vi "Advanced Serial Write and Read - Black Magic Voodo.vi"(0 "VISA resource name":refnum<visa-resource-name>="COM11", 13 "string to write":string="*IDN?", 17 "write":bool=TRUE, 26 "read":bool=TRUE) -> (20 "read string":string)   [LabVIEW 2010]
doc: "The Advanced Serial Read and Write example performs a Serial Port Read, a Serial Port Write, or a combination of these actions while setting some advanced serial features like buffer size, termination characters, and XON/XOFF flow control. The user selects the actions (read or write) on the front panel. If both are selected, the VI will write the data first, read the data and then close the VISA session that is opened to the port. \n\nThe parameters set for the serial port must match the parameters of the connected instrument or device. In this example, the bytes to read parameter specifies the number of bytes that the serial port reads. If there were more bytes at the port than the number specified in bytes to read, those bytes would not be read. Also, if you specify to read more bytes than the number of bytes actually read, you might receive a timeout error message.\n\nINSTRUCTIONS:\n1) Select the serial resource and configuration parameters (baud rate, data bits, parity, stop bits, flow control).\n2) Termination character can be enabled and set. Also, set the required input buffer size prior to running the example.\n3) Select the operations to be performed. \n4) Connect the serial port to your device. If no device is available, perform a loopback test by doing one of the following. Short pins 2 and 3 on a RS-232 cable or short pin 4 to pin 8 and pin 5 to pin 9 on a RS-485/422 cable. \n5) Run the VI to see the data read. (The \"read string\" will match the \"string to write\" if a loopback test was performed.)\n\nThis example exposes several advanced features that you may need for your application. Not all applications need all the features shown in this example. The input buffer size is likely an important setting that you want to control in your application. This example expands upon the flow control option for XON and XOFF, allowing the user to choose those control characters. The timeout parameter has been brought to the front panel so a user can specify the time period the VISA Read will wait for the number of bytes to read before timing out. Also, the user has several controls for the termination character, which is discussed later.\n\nNote that you can press the write and read buttons and change the bytes to read parameters on the fly, while the example is running. However, you must stop the example to change the other configuration parameters after the example has started running, and then run again.\n\nSet the I/O buffer size slightly higher the amount of data you expect to receive. This is very important for applications that don't use flow control, as you may lose characters if the receive buffer overflows.\n\nSetting the timeout period ensures that the operation returns with a timeout error if the operation cannot be performed in the specified time period. \n\nSome devices require a termination character in order to identify the end of command strings. Some devices send a termination character to signify the end of data to be read. \n\nThis example shows how you can end the Read operation once a termination character is detected in the buffer and/or append a termination character at the end of the Write data. To enable the Read to end on a termination character, use the VISA Configure Serial Port or use the VISA Properties Serial End Mode for Reads, Termination Character Enable, and Termination Character. To end the Write with a termination character, use the VISA Properties Serial End Mode for Writes, the Send End Enable, and Termination Character. In this example, the same termination character is used for both the Read and the Write. You can specify two different characters for your application, if desired.\n\nYour application may require specific characters for the XON/XOFF Flow Control. You can specify these characters with the VISA Properties Flow Control XOFF Character and Flow Control XON Character. Note that if the standard XON and XOFF characters are used, then decimal 17 and 19 are unavailable for data values. Remember that using flow control and setting an adequate buffer size allow you to prevent buffer overflows."
uses:
  <vilib>/Instr/_visa.llb/VISA Configure Serial Port (Instr).vi
panel:
  in  "String":string="(RS232(Sources (\"CO2B um/m\" \"H2OB mm/m\"  \"Integral\" \"Peak\" \"P kPa\" \"T C\" ))) "
  out "iteration":dbl
  out "actual bytes read":u32
  in  "stop":bool
  # "Select the serial resource and the operations to be performed.  If all are selected, the VI will write the data first, read data and then close the VISA session that is opened to the port.  This VI will wait until the specified number of bytes is received at the port, until the timeout period is met, or until a termination character is received.  The default termination character in this example is the Line Feed ( ASCII 0xA, '\\n' ).  Also, set the required input buffer size prior to running the example.\nNote: The example loops until the STOP button is pressed."
  # "For additional information select File >> VI Properties >> Documentation"
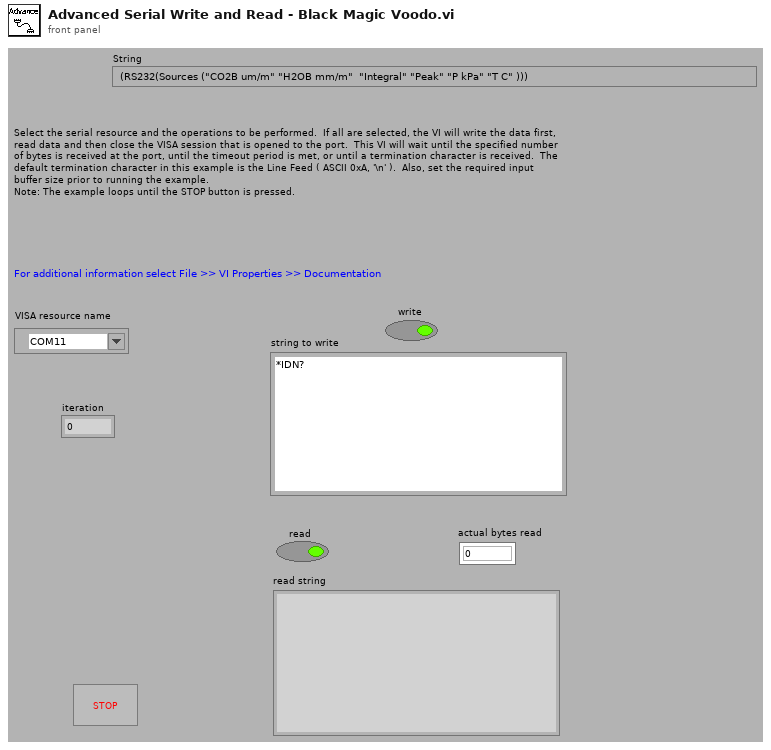
[diagram p1: front panel]
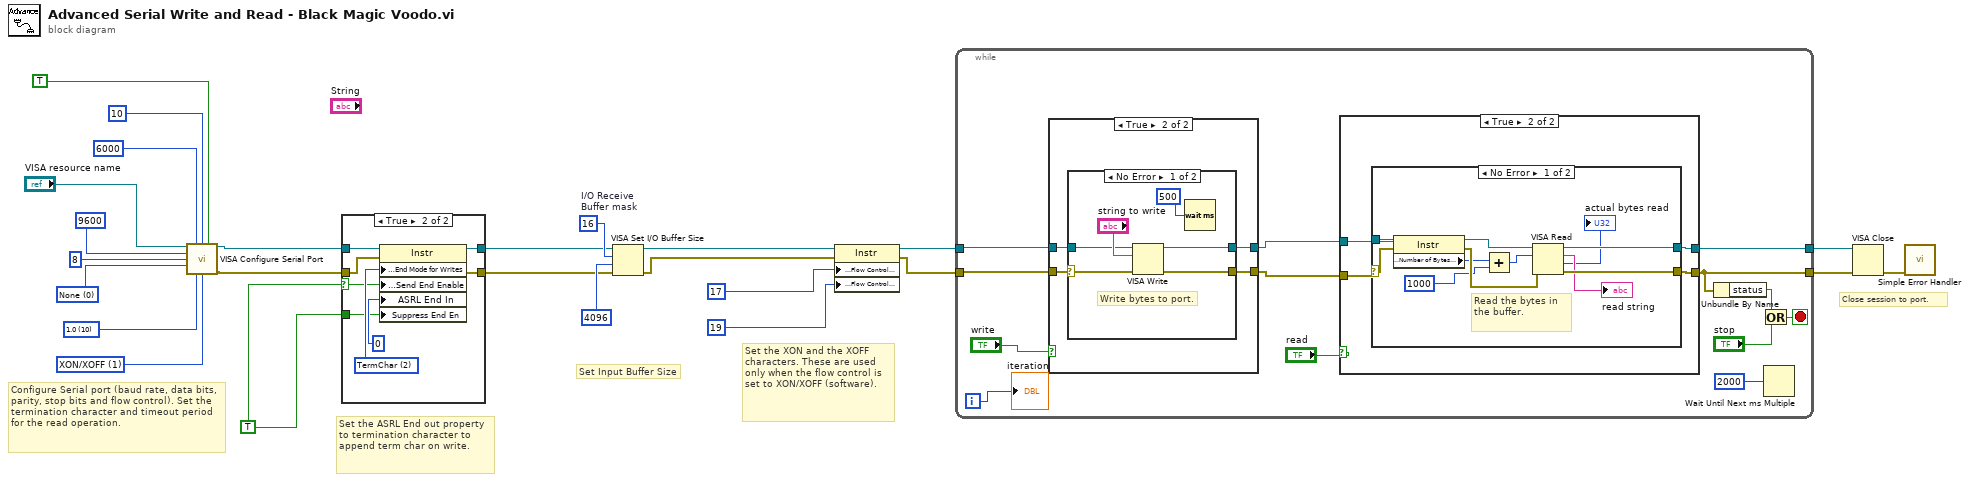
[diagram p0: block diagram]
diagram:
  w1 = TRUE ("End write with termination character?")
  w15 = u16 1 items=["None"=0, "XON/XOFF"=1, "RTS/CTS"=2, "DTR/DSR"=4] ("flow control")
  w21 = u16 10 items=["1.0"=10, "1.5"=15, "2.0"=20] ("stop bits")
  w22 = u16 0 items=["None", "Odd", "Even", "Mark", "Space"] ("parity")
  w18 = u16 16  # I/O Receive Buffer mask
  # "Set the XON and the XOFF characters. These are used only when the flow control is set to XON/XOFF (software)."
  # "Configure Serial port (baud rate, data bits, parity, stop bits and flow control). Set the termination character and timeout period for the read operation."
  # "Set Input Buffer Size"
  # "Set the ASRL End out property to termination character to append term char on write."
  # "Close session to port."
  n1 = call-poly "VISA Configure Serial Port"("VISA resource name"="VISA resource name", "timeout (10sec)"=u32 6000 ("timeout (ms)"), "termination char\n(0xA = '\\n' = LF)"=u8 10 ("termination char\n(0xA = '\\n' = LF)"), "Enable Termination\nChar (T)"=TRUE ("End read on termination character?"), "baud rate (9600)"=u32 9600 ("baud rate"), "data bits (8)"=u16 8 ("data bits"), "parity (0:none)"=w22, "stop bits (10: 1 bit)"=w21, "flow control (0:none)"=w15) -> ("VISA resource name out"=w3:refnum<visa-resource-name>, "error out"=w2:errorcluster)  [unwired: 1 in, 4 out]
  n2 = case shown="True" w1 {
    selector: w1 -> [_ w30]
    tunnel: w3 -> [w26 w35]
    tunnel: w2 -> [w27 w34]
    tunnel: [w26 w33] -> w7
    tunnel: [w27 w32] -> w8
    tunnel: w1 -> [_ w28]
    frame False {
    }
    frame True {
      w31 = u16 2 items=["None", "LastBit", "TermChar", "Break"] ("Serial Settings:Serial End Mode for Writes")
      n3 = property class="Instr"(reference=w35, error in=w34, "Serial Settings:End Mode for Writes"=w31, "Message Based Settings:Send End Enable"=w30, "ASRL End In"=0, "Suppress End En"=w28) -> (reference out=w33:refnum<visa-resource-name>, error out=w32:errorcluster)
    }
  }
  n4 = VISA Set I/O Buffer Size(VISA resource name=w7, mask (16)=w18, size (4096)=u32 4096 ("Input\nbuffer size"), error in (no error)=w8) -> (VISA resource name out=w14:refnum<visa-resource-name>, error out=w13:errorcluster)
  n5 = property class="Instr"(reference=w14, error in=w13, "Serial Settings:Flow Control XON Character"=u8 17 ("XON Character"), "Serial Settings:Flow Control XOFF Character"=u8 19 ("XOFF Character")) -> (reference out=w6:refnum<visa-resource-name>, error out=w10:errorcluster)
  n6 = while {
    tunnel: w10 -> [w43]
    tunnel: w6 -> [w44]
    tunnel: [w42] -> w5
    tunnel: [w41] -> w4
    i -> [w36]
    stop <- w40 stop-if-true
    n7 = case shown="True" "write" {
      tunnel: [w50 w54] -> w38
      tunnel: [w49 w53] -> w37
      tunnel: w44 -> [w50 w52]
      tunnel: w43 -> [w49 w51]
      frame False {
      }
      frame True {
        n8 = case shown="No Error" w51 {
          selector: w51 -> [w56 w62]
          tunnel: [w60 w61] -> w54
          tunnel: [w59 w62] -> w53
          tunnel: w52 -> [w57 w61]
          frame No Error {
            # "Write bytes to port."
            n9 = VISA Write(VISA resource name=w57, write buffer="string to write", error in (no error)=w56) -> (VISA resource name out=w60:refnum<visa-resource-name>, error out=w59:errorcluster)  [unwired: 1 out]
            n10 = Wait (ms)(milliseconds to wait=500) -> ()  [unwired: 1 out]
          }
          frame Error {
          }
        }
      }
    }
    n11 = case shown="True" "read" {
      tunnel: [w64 w68] -> w41
      tunnel: [w63 w67] -> w42
      tunnel: w37 -> [w64 w66]
      tunnel: w38 -> [w63 w65]
      frame False {
      }
      frame True {
        n12 = case "Read bytes from port." shown="No Error" w66 {
          selector: w66 -> [w74 w81]
          tunnel: [w78 w81] -> w68
          tunnel: [w79 w80] -> w67
          tunnel: w65 -> [w75 w80]
          frame No Error {
            # "Read the bytes in the buffer."
            n13 = property class="Instr"(reference=w75, error in=w74) -> (reference out=w73:refnum<visa-resource-name>, error out=w72:errorcluster, "Serial Settings:Number of Bytes at Serial Port"=w71:u32)
            n14 = Add(x=w71, y=1000) -> (x+y=w70:u32)
            n15 = VISA Read(VISA resource name=w73, byte count=w70, error in (no error)=w72) -> (VISA resource name out=w79:refnum<visa-resource-name>, read buffer=→"read string":string, return count=→"actual bytes read":u32, error out=w78:errorcluster)
          }
          frame Error {
            # "Error occurred \nreading Bytes at \nSerial Port"
          }
        }
      }
    }
    n16 = Unbundle By Name(w41) -> ("status"=w46:bool)
    n17 = Or(x=w46, y="stop") -> (x .or. y?=w40:bool)
    n18 = Wait Until Next ms Multiple(millisecond multiple=u32 2000) -> ()  [unwired: 1 out]
    "iteration" <- w36
  }
  n19 = VISA Close(VISA resource name=w5, error in (no error)=w4) -> (error out=w23:errorcluster)
  n20 = call <vilib>:"Simple Error Handler.vi"("error in (no error)"=w23) -> ()  [unwired: 1 in, 8 out]
